vi "user output.vi"(8 "error in":errorcluster, 11 "Outputs to system":T1) -> (0 "error out":errorcluster)   [LabVIEW 2017, in "Convert Bool to Velocity runtime.lvclass"]
uses:
  Convert Bool to Velocity runtime.lvclass
  output user data.ctl
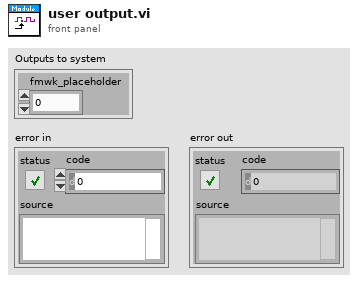
[diagram p1: front panel]
types:
  T1 = typedef "Convert Bool to Velocity runtime.lvclass/output user data.ctl" = cluster{"fmwk_placeholder":i32}
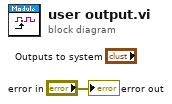
[diagram p0: block diagram]
diagram:
  "error out" <- "error in"
